vi "DeMux1.vi"(2 "X":bool, 3 "S":bool) -> (0 "B":bool, 1 "A":bool)   [LabVIEW 2012]
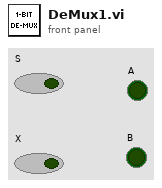
[diagram p1: front panel]
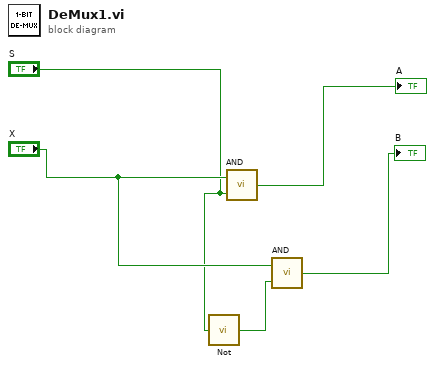
[diagram p0: block diagram]
diagram:
  n1 = call "Not.vi"("In"="S") -> ("Out"=w2:bool)
  n2 = call "AND.vi"("b"="S", "a"="X") -> ("x"=→"A":bool)
  n3 = call "AND.vi"("b"=w2, "a"="X") -> ("x"=→"B":bool)
